vi "Write Rolebook.vi"(8 "error in (no error)":errorcluster, 10 "Rolebook":refnum<class "Rolebook.lvclass">, 11 "Play in":refnum<class "Play.lvclass">) -> (0 "error out":errorcluster, 3 "Play out":refnum<class "Play.lvclass">)   [LabVIEW 2023, in "Play.lvclass"]
uses:
  Play.lvclass
  Rolebook_class/Rolebook.lvclass
  Play.lvclass/Play.ctl
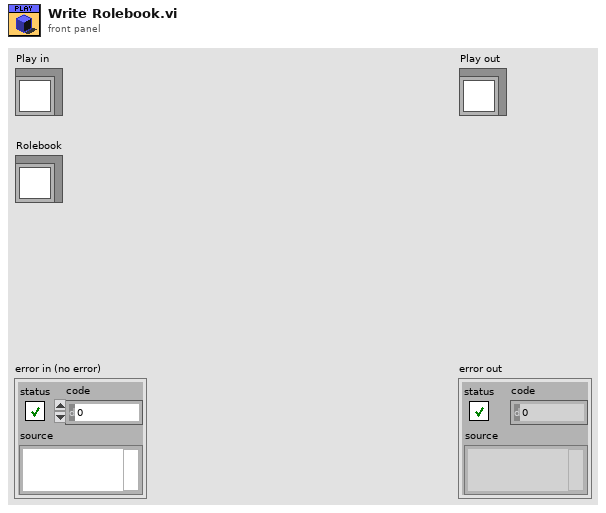
[diagram p1: front panel]
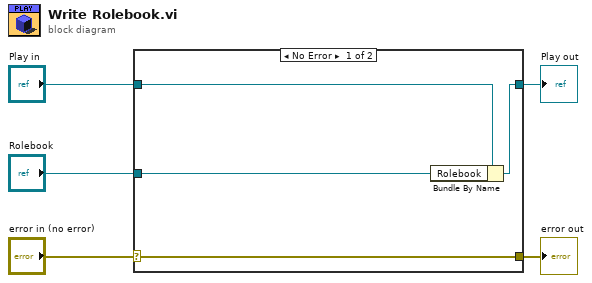
[diagram p0: block diagram]
diagram:
  n1 = case shown="No Error" "error in (no error)" {
    selector: "error in (no error)" -> [w9 w10]
    tunnel: [w9 w10] -> w4
    tunnel: [w7 w11] -> w2
    tunnel: "Play in" -> [w8 w11]
    tunnel: "Rolebook" -> [w6 _]
    frame No Error {
      n2 = Bundle By Name(cluster=w8, "Rolebook"=w6) -> (w7:refnum<class "Play.lvclass">)
    }
    frame Error {
    }
  }
  "error out" <- w4
  "Play out" <- w2
